vi "KMAX Spectrometer 1.0.vi"() -> ()   [LabVIEW 2023]
uses:
  <vilib>/userDefined/High Color/IMAQdx.ctl
  <vilib>/Utility/file.llb/Read Delimited Spreadsheet (DBL).vi
  <vilib>/Utility/file.llb/Write Delimited Spreadsheet (DBL).vi
panel:
  in  "Integration Time (ms)":dbl=5.0 min=5.0 max=1000.0 step=1.0
  in  "error in (no error)":errorcluster
  in  "Camera Name":T1
  in  "Averaging":bool
  out "Completed":i32
  in  "Averages":i32=1 min=1 max=100
  in  "Autoscale Vertical Axis":bool=TRUE
  in  "Subtract Background":bool
  in  "Take Background?":bool
  in  "Load?":bool
  in  "OK Button":bool
  out "Message":string
  out "FWHM":dbl
  in  "Save?":bool
  out "Spectra":cluster{"all rows":dbl[], "all rows":dbl[]}[](graph)
  in  "Stop":bool
  # "nm"
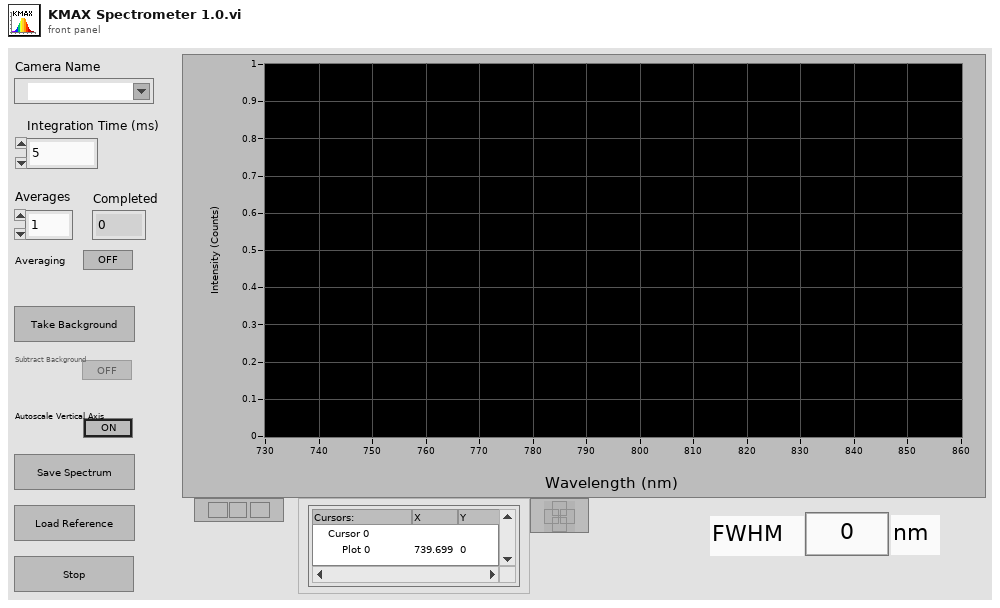
[diagram p1: front panel]
types:
  T1 = typedef "IMAQdx.ctl" = refnum<k21>
  T2 = enum8{"Enabled", "Disabled", "Disabled and Grayed Out"}
  T3 = typedef "IMAQ Image.ctl" = refnum<image>
  T4 = cluster{"Wavelengths (nm)":dbl[], "Intensity":dbl[]}
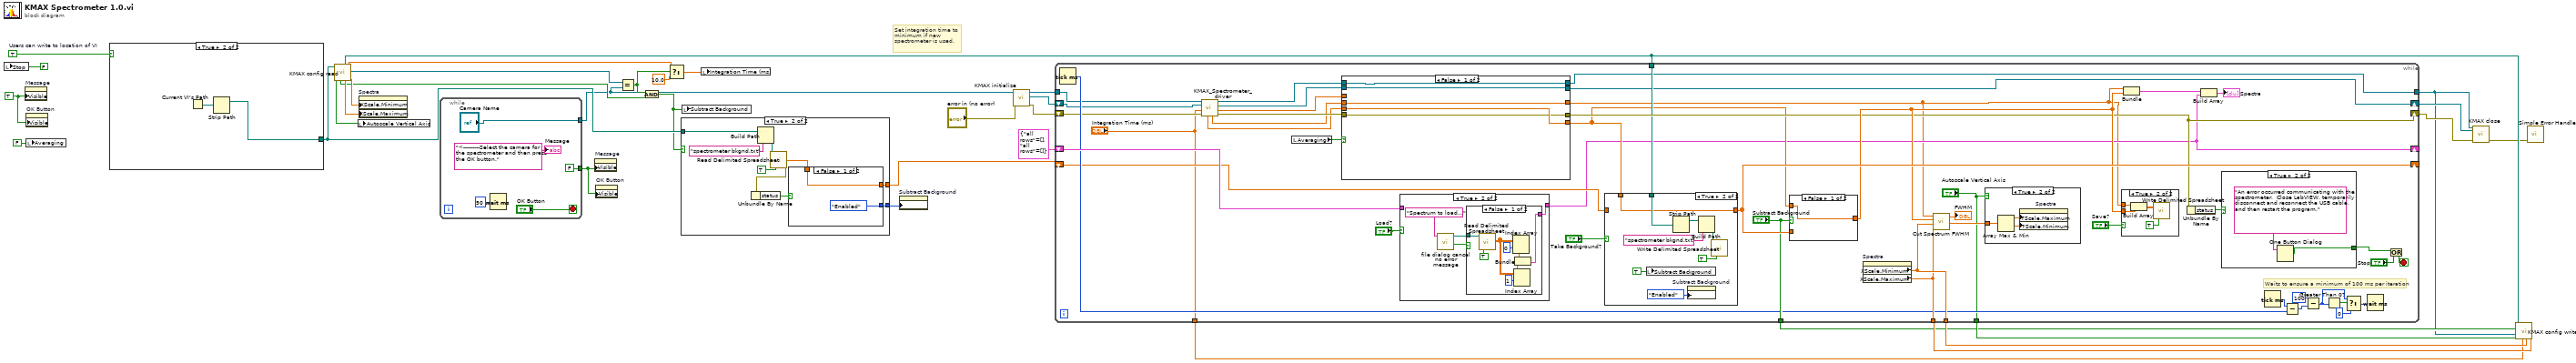
[diagram p0: block diagram]
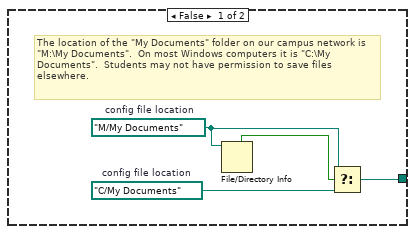
[diagram p2: hidden frame]
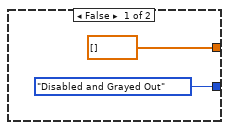
[diagram p3: hidden frame]
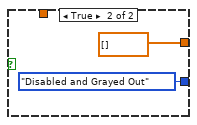
[diagram p4: hidden frame]
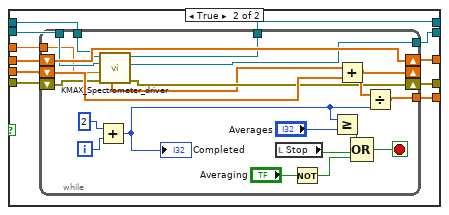
[diagram p5: hidden frame]
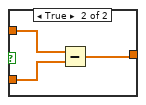
[diagram p7: hidden frame]
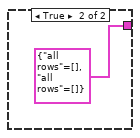
[diagram p10: hidden frame]
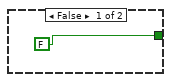
[diagram p11: hidden frame]
diagram:
  w19 = TRUE  # Users can write to location of VI
  w32 = TRUE ("Visible")
  # "Set integration time to minimum if new spectrometer is used."
  n1 = local write "Stop"(FALSE ("Stop")) -> ()
  n2 = property on="Message" class="Str"("Visible"=w32) -> ()  [unwired: 2 in, 2 out]
  n3 = property on="OK Button" class="Bool"("Visible"=w32) -> ()  [unwired: 2 in, 2 out]
  n4 = local write "Averaging"(FALSE ("Averaging")) -> ()
  n5 = case shown="True" w19 {
    tunnel: [w35 w39] -> w20
    frame False {
      w37 = path "C:/My Documents"  # config file location
      w36 = path "M:/My Documents"  # config file location
      # "The location of the \"My Documents\" folder on our campus network is \"M:\\My Documents\".  On most Windows computers it is \"C:\\My Documents\".  Students may not have permission to save files elsewhere."
      n6 = File/Directory Info(path=w36) -> (directory=w38:bool)  [unwired: 1 in, 6 out]
      n7 = Select(t=w36, s=w38, f=w37) -> (s? t:f=w35:path)
    }
    frame True {
      n8 = Current VI's Path() -> (path=w40:path)
      n9 = Strip Path(path=w40) -> (stripped path=w39:path)  [unwired: 1 out]
    }
  }
  n10 = call "KMAX config read.vi"("config file location"=w20) -> ("XScale.Minimum"=w31:dbl, "Integration Time (5 ms)"=w15:dbl, "Camera Name"=w12:refnum<k21>, "XScale.Maximum"=w30:dbl, "configuration file path"=w21:path, "Background"=w18:bool, "Autoscale"=w24:bool)  [unwired: 4 in]
  n11 = local write "Autoscale Vertical Axis"(w24) -> ()
  n12 = property on="Spectra" class="XYGraph (strict)"("XScale.Minimum"=w31, "XScale.Maximum"=w30) -> ()  [unwired: 2 in, 2 out]
  n13 = while {
    tunnel: ["Camera Name"] -> w9
    tunnel: [FALSE ("Stop")] -> w33
    stop <- "OK Button" stop-if-true
    n14 = Wait (ms)(milliseconds to wait=u32 50 ("millisecond multiple")) -> ()  [unwired: 1 out]
    "Message" <- "<---------Select the camera for the spectrometer and then press the OK button." ("Message")
  }
  n15 = property on="Message" class="Str"("Visible"=w33) -> ()  [unwired: 2 in, 2 out]
  n16 = property on="OK Button" class="Bool"("Visible"=w33) -> ()  [unwired: 2 in, 2 out]
  n17 = Equal?(x=w12, y=w9) -> (x = y?=w17:bool)
  n18 = And(x=w17, y=w18) -> (x .and. y?=w16:bool)
  n19 = Select(t=w15, s=w17, f=10.0 ("t")) -> (s? t:f=w2:dbl)
  n20 = case shown="True" w16 {
    tunnel: [dbl[] [] ("first row") w51] -> w23
    tunnel: [T2."Disabled and Grayed Out" ("Disabled") w50] -> w22
    tunnel: w20 -> [_ w48]
    frame False {
    }
    frame True {
      n21 = Build Path(base path=w48, name or relative path="spectrometer bkgnd.txt") -> (appended path=w55:path)
      n22 = call-poly <vilib>:"Read Delimited Spreadsheet.vi"("file path (dialog if empty)"=w55, "transpose? (F)"=TRUE ("transpose? (no:F)")) -> ("first row"=w49:dbl[], "error out"=w53:errorcluster)  [unwired: 8 in, 4 out]
      n23 = Unbundle By Name(w53) -> ("status"=w52:bool)
      n24 = case shown="False" w52 {
        tunnel: [w57 dbl[] [] ("first row")] -> w51
        tunnel: [T2."Enabled" ("Disabled") T2."Disabled and Grayed Out" ("Disabled")] -> w50
        tunnel: w49 -> [w57 _]
        frame False {
        }
        frame True {
        }
      }
    }
  }
  n25 = local write "Subtract Background"(w16) -> ()
  n26 = local write "Integration Time (ms)"(w2) -> ()
  n27 = property on="Subtract Background" class="Bool (strict)"("DisabledEnum"=w22) -> ()  [unwired: 2 in, 2 out]
  n28 = call "KMAX initialize.vi"("error in (no error)"="error in (no error)", "Refnum in"=w9) -> ("error out"=w7:errorcluster, "New Image"=w8:T3, "Refnum out"=w5:T1)  [unwired: 7 in]
  n29 = while {
    shift-right: [w92] -> w11
    shift-left: w7 -> [w74]
    shift-right: [w76] -> _
    shift-left: cluster{"all rows":dbl[], "all rows":dbl[]} {"all rows"=[], "all rows"=[]} -> [w99]
    shift-right: [w96] -> _
    shift-left: w23 -> [w77]
    tunnel: [w94] -> w29
    tunnel: [w93] -> w28
    tunnel: ["Autoscale Vertical Axis"] -> w26
    tunnel: ["Subtract Background"] -> w25
    tunnel: w21 -> [w90]
    shift-right: [w65] -> w4
    shift-left: w8 -> [w72]
    tunnel: w5 -> [w64]
    tunnel: [w63] -> w3
    tunnel: ["Integration Time (ms)"] -> w1
    stop <- w102 stop-if-true
    # "Waits to ensure a minimum of 100 ms per iteration"
    n30 = Tick Count (ms)() -> (millisecond timer value=w82:u32)
    n31 = call "KMAX_Spectrometer_driver.vi"("error in"=w74, "IntegrationTime (ms)"="Integration Time (ms)", "New Image"=w72, "Camera Name"=w64) -> ("error out"=w73:errorcluster, "Integration Time Output (ms)"=w62:dbl, "Image Out"=w68:T3, "Session Out"=w69:T1, "Wavelengths (nm)"=w71:dbl[], "Intensity"=w70:sgl[])  [unwired: 2 in]
    n32 = local read "Averaging"() -> (w75:bool)
    n33 = case shown="False" w75 {
      tunnel: [w108 w121] -> w66
      tunnel: [w109 w120] -> w92
      tunnel: [w110 w119] -> w78
      tunnel: w73 -> [w109 w118]
      tunnel: w70 -> [w110 w117]
      tunnel: w62 -> [_ w116]
      tunnel: w71 -> [w108 w115]
      tunnel: w69 -> [w107 w114]
      tunnel: w68 -> [w106 w113]
      tunnel: [w107 w112] -> w63
      tunnel: [w106 w111] -> w65
      frame False {
      }
      frame True {
        n34 = while {
          shift-right: [w128] -> w121
          shift-left: w115 -> [w128]
          shift-right: [w129] -> w120
          shift-left: w118 -> [w130]
          shift-right: [w138] -> _
          shift-left: w117 -> [w139]
          tunnel: [w137] -> w119
          tunnel: w116 -> [w125]
          tunnel: w114 -> [w127]
          tunnel: w113 -> [w126]
          tunnel: [w123] -> w112
          tunnel: [w122] -> w111
          i -> [w136]
          stop <- w140 stop-if-true
          n35 = Add(x=2, y=w136) -> (x+y=w132:i32)
          "Completed" <- w132
          n36 = call "KMAX_Spectrometer_driver.vi"("error in"=w130, "IntegrationTime (ms)"=w125, "New Image"=w126, "Camera Name"=w127) -> ("error out"=w129:errorcluster, "Image Out"=w122:T3, "Session Out"=w123:T1, "Intensity"=w124:sgl[])  [unwired: 2 in, 2 out]
          n37 = local read "Stop"() -> (w141:bool)
          n38 = Not(x="Averaging") -> (.not. x?=w133:bool)
          n39 = Greater Or Equal?(x=w132, y="Averages") -> (x >= y?=w142:bool)
          n40 = Add(x=w124, y=w139) -> (x+y=w138:sgl[])
          n41 = Compound Arithmetic op=OR(w142, w141, w133) -> (w140:bool)
          n42 = Divide(x=w138, y=w132) -> (x/y=w137:sgl[])
        }
      }
    }
    n43 = case shown="True" "Load?" {
      tunnel: [w159 w163] -> w76
      tunnel: w99 -> [w159 _]
      frame False {
      }
      frame True {
        n44 = call "file dialog cancel no error message.vi"("prompt"="Spectrum to load...") -> ("cancelled"=w161:bool, "path"=w160:path)  [unwired: 9 in]
        n45 = case shown="False" w161 {
          tunnel: [w165 cluster{"all rows":dbl[], "all rows":dbl[]} {"all rows"=[], "all rows"=[]}] -> w163
          tunnel: w160 -> [w164 _]
          frame False {
            n46 = call-poly <vilib>:"Read Delimited Spreadsheet.vi"("file path (dialog if empty)"=w164, "transpose? (F)"=TRUE) -> ("all rows"=w168:dbl[][])  [unwired: 8 in, 5 out]
            n47 = Index Array(array=w168, index (row)=0) -> (element=w167:dbl[])  [unwired: 1 in]
            n48 = Index Array(array=w168, index (row)=1) -> (element=w166:dbl[])  [unwired: 1 in]
            n49 = Bundle("all rows"=w167, "all rows"=w166) -> (w165:cluster{"all rows":dbl[], "all rows":dbl[]})  [unwired: 1 in]
          }
          frame True {
          }
        }
      }
    }
    n50 = case shown="True" "Take Background?" {
      tunnel: w78 -> [_ w151]
      tunnel: [w150 w151] -> w96
      tunnel: w77 -> [w150 _]
      tunnel: w90 -> [_ w152]
      frame False {
      }
      frame True {
        n51 = local write "Subtract Background"(TRUE ("Subtract Background")) -> ()
        n52 = Strip Path(path=w152) -> (stripped path=w153:path)  [unwired: 1 out]
        n53 = property on="Subtract Background" class="Bool (strict)"("DisabledEnum"=T2."Enabled" ("Disabled")) -> ()  [unwired: 2 in, 2 out]
        n54 = Build Path(base path=w153, name or relative path="spectrometer bkgnd.txt") -> (appended path=w155:path)
        n55 = call-poly <vilib>:"Write Delimited Spreadsheet.vi"("file path (dialog if empty)"=w155, "transpose? (no:F)"=TRUE) -> ()  [unwired: 12 in, 2 out]
      }
    }
    n56 = case shown="False" "Subtract Background" {
      tunnel: w78 -> [w146 w149]
      tunnel: w96 -> [_ w148]
      tunnel: [w146 w147] -> w95
      frame False {
      }
      frame True {
        n57 = Subtract(x=w149, y=w148) -> (x-y=w147:dbl[])
      }
    }
    n58 = property on="Spectra" class="XYGraph (strict)"() -> ("XScale.Minimum"=w94:dbl, "XScale.Maximum"=w93:dbl)  [unwired: 2 in, 2 out]
    n59 = call "Cut Spectrum FWHM.vi"("XScale.Maximum"=w93, "XScale.Minimum"=w94, "Intensities"=w95, "Wavelengths"=w66) -> ("Cut Intensities"=w81:dbl[], "FWHM"=→"FWHM":dbl)
    n60 = case shown="True" "Autoscale Vertical Axis" {
      tunnel: w81 -> [_ w143]
      frame False {
      }
      frame True {
        n61 = Array Max & Min(array=w143) -> (max value=w145:dbl, min value=w144:dbl)  [unwired: 2 out]
        n62 = property on="Spectra" class="XYGraph (strict)"("YScale.Maximum"=w145, "YScale.Minimum"=w144) -> ()  [unwired: 2 in, 2 out]
      }
    }
    n63 = case shown="True" "Save?" {
      tunnel: w95 -> [_ w179]
      tunnel: w66 -> [_ w176]
      frame False {
      }
      frame True {
        n64 = Build Array(w176, w179) -> (w178:dbl[][])
        n65 = call-poly <vilib>:"Write Delimited Spreadsheet.vi"("2D data"=w178, "transpose? (no:F)"=TRUE) -> ()  [unwired: 12 in, 2 out]
      }
    }
    n66 = Bundle("Wavelengths (nm)"=w66, "Intensity"=w95) -> (w67:T4)  [unwired: 1 out]
    n67 = Unbundle By Name(w92) -> ("status"=w104:bool)
    n68 = Build Array(w67, w76) -> (→"Spectra":cluster{"all rows":dbl[], "all rows":dbl[]}[])
    n69 = case shown="True" w104 {
      tunnel: [FALSE ("true") w174] -> w101
      frame False {
      }
      frame True {
        n70 = One Button Dialog(message="An error occurred communicating with the spectrometer.  Close LabVIEW, temporarily disconnect and reconnect the USB cable, and then restart the program.") -> (true=w174:bool)  [unwired: 1 in]
      }
    }
    n71 = Tick Count (ms)() -> (millisecond timer value=w89:u32)
    n72 = Subtract(x=w89, y=w82) -> (x-y=w88:u32)
    n73 = Subtract(x=u32 100, y=w88) -> (x-y=w85:u32)
    n74 = Greater Than 0?(x=w85) -> (x > 0?=w86:bool)
    n75 = Select(t=w85, s=w86, f=u32 0) -> (s? t:f=w83:u32)
    n76 = Wait (ms)(milliseconds to wait=w83) -> ()  [unwired: 1 out]
    n77 = Or(x=w101, y="Stop") -> (x .or. y?=w102:bool)
  }
  n78 = call "KMAX close.vi"("error in (no error)"=w11, "Image Out"=w4, "Refnum in"=w3) -> ("error out"=w10:errorcluster)  [unwired: 8 in]
  n79 = call "KMAX config write.vi"("XScale.Maximum"=w28, "XScale.Minimum"=w29, "Integration Time (5 ms)"=w1, "Autoscale"=w26, "Camera Name"=w3, "Background"=w25, "configuration file path"=w21) -> ()  [unwired: 5 in]
  n80 = call <vilib>:"Simple Error Handler.vi"("error in (no error)"=w10) -> ()  [unwired: 1 in, 8 out]
